vi "Set Run Mode.vi"(8 "error in (no error)":errorcluster, 10 "Run Control":T1, 11 "VISA resource name":refnum<visa-resource-name>) -> (0 "error out":errorcluster, 3 "VISA resource name out":refnum<visa-resource-name>)   [LabVIEW 2018, in "DPO4104.lvlib" / "DPO4104.lvclass"]
doc: "This VI sends commands for Run (Continuous), Single and Stop operation."
uses:
  DPO4104.lvclass
  PPLs/Oscilloscope/Parent/Oscilloscope.lvlibp/Custom Controls/Run Control.ctl
  <instrlib>/Tektronix DPO MSO 2000 4000 Series/Tektronix DPO MSO 2000 4000 Series.lvlib
  PPLs/Oscilloscope/Parent/Oscilloscope.lvlibp
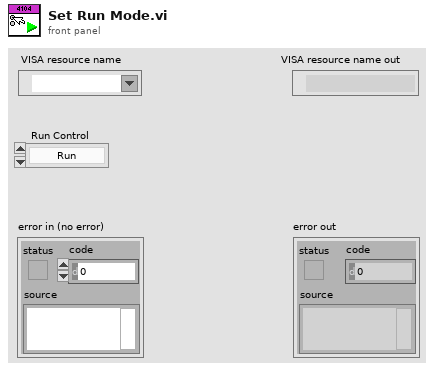
[diagram p1: front panel]
types:
  T1 = typedef "Oscilloscope.lvlibp/Run Control.ctl" = enum16{"Run", "Single", "Stop"}
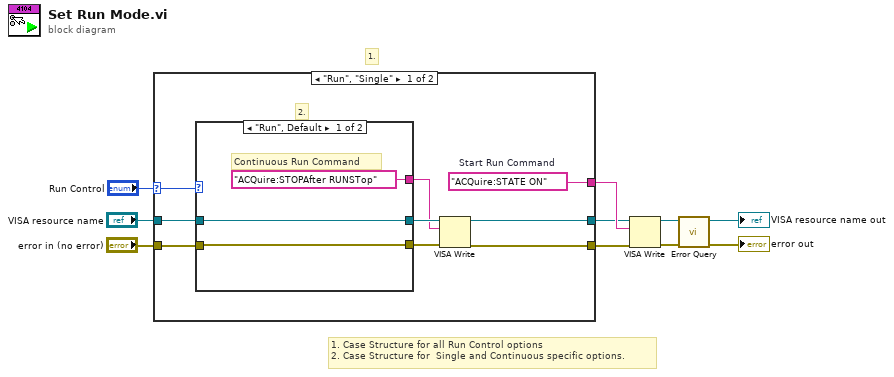
[diagram p0: block diagram]
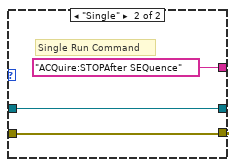
[diagram p2: hidden frame]
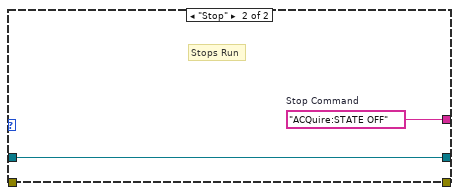
[diagram p3: hidden frame]
diagram:
  # "1. Case Structure for all Run Control options\n2. Case Structure for  Single and Continuous specific options."
  # "1."
  n1 = case shown="\"Run\", \"Single\"" "Run Control" {
    selector: "Run Control" -> [w19 _]
    tunnel: [w13 w27] -> w5
    tunnel: [w12 w26] -> w3
    tunnel: "VISA resource name" -> [w16 w26]
    tunnel: [w11 _] -> w1
    tunnel: "error in (no error)" -> [w18 _]
    frame "Run", "Single" {
      w13 = "ACQuire:STATE ON"  # Start Run Command
      # "2."
      n2 = case shown="\"Run\", Default" w19 {
        tunnel: [w21 w25] -> w17
        tunnel: w18 -> [w21 w25]
        tunnel: [w22 w24] -> w15
        tunnel: w16 -> [w22 w24]
        tunnel: ["ACQuire:STOPAfter RUNSTop" "ACQuire:STOPAfter SEQuence"] -> w14
        frame "Run", Default {
          # "Continuous Run Command"
        }
        frame "Single" {
          # "Single Run Command"
        }
      }
      n3 = VISA Write(VISA resource name=w15, write buffer=w14, error in (no error)=w17) -> (VISA resource name out=w12:refnum<visa-resource-name>, error out=w11:errorcluster)  [unwired: 1 out]
    }
    frame "Stop" {
      w27 = "ACQuire:STATE OFF"  # Stop Command
      # "Stops Run"
    }
  }
  n4 = VISA Write(VISA resource name=w3, write buffer=w5, error in (no error)=w1) -> (VISA resource name out=w7:refnum<visa-resource-name>, error out=w6:errorcluster)  [unwired: 1 out]
  n5 = call <instrlib>:"Error Query.vi"("error in (no error)"=w6, "VISA resource name"=w7) -> ("error out"=→"error out":errorcluster, "VISA resource name out"=→"VISA resource name out":refnum<visa-resource-name>)  [unwired: 6 in, 2 out]
